vi "Log SPAN autorun Errors.vi"(3 "CompSep":bool, 4 "Sprachliste":string[][](array[string]), 5 "Gasteiler Type":T4 items=["LNI", "Analog-Display", "AVL GDU", "Horiba GDC", "HovaCal", "Horiba SGD 710C"], 6 "Component Infos":T1, 7 "LogFileName_Präfix":string="AutoSpanLin_ErrorLog_", 8 "error in (no error)":errorcluster caption="Fehler (Eingang, kein Fehler)", 9 "LogInfo-Einstellung-Cluster":T5, 10 "LogInfo-Cluster":T6 {"Gasflasche" items=["----"=10000, "IAG NH3 3000"=0, "IAG NH3 200"=1, "IAG NH3 2000"=2, "IAG MG"=3, "IAG O2"=4]}, 11 "Pfad LIN":T8 caption="Pfad") -> (0 "error out":errorcluster caption="Fehler (Ausgang)")   [LabVIEW 2020, in "Linearisierung v2.lvlib" / "SpanEinstellungen.lvlib"]
uses:
  SpanEinstellungen.lvlib
  Visualisierungs Elemente/Pfad-Eingabefeld.ctl
  ErrorLogInfoCluster.ctl
  Visualisierungs Elemente/String - Ausgabefeld.ctl
  Seiten/System Einstellungen V2/Gasflasche Auswahl.ctl
  GasteilerType.ctl
  ComponentInfos.ctl
  Visualisierungs Elemente/String - Eingabefeld.ctl
  Seiten/System Einstellungen V2/Aktion FGV Gasbottledefinition.ctl
  Gasteiler/Aktionen FGV Gasteiler Daten.ctl
  Seiten/System Einstellungen V2/System Einstellungen V2.lvlib
  Gasteiler/Gasteiler.lvlib
  Sprachverwaltung/Sprachverwaltung.lvlib
  Protokoll/Protokoll.lvlib
  Linearisierung v2.lvlib
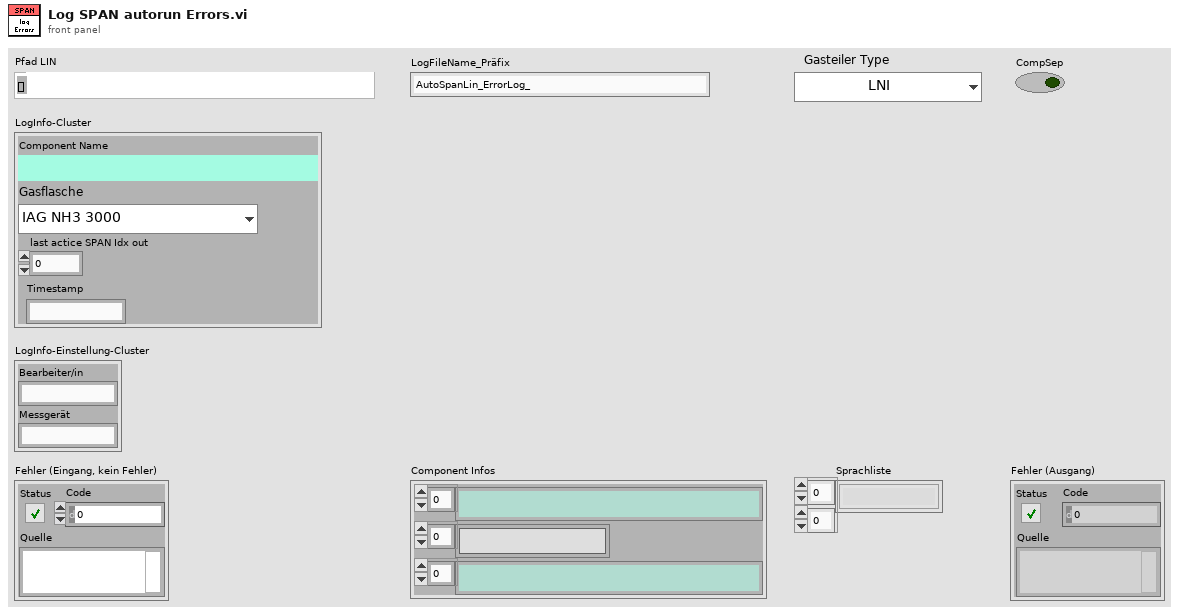
[diagram p1: front panel]
types:
  T1 = typedef "Linearisierung v2.lvlib/SpanEinstellungen.lvlib/ComponentInfos.ctl" = cluster{T2[], T3[], T2[]}
  T2 = typedef "String - Ausgabefeld.ctl" = string
  T3 = typedef "String - Eingabefeld.ctl" = string
  T4 = typedef "Linearisierung v2.lvlib/GasteilerType.ctl" = u16
  T5 = cluster{"Bearbeiter/in":string, "Messgerät":string}
  T6 = typedef "Linearisierung v2.lvlib/SpanEinstellungen.lvlib/ErrorLogInfoCluster.ctl" = cluster{"Component Name":T2, "Gasflasche":T7, "last actice SPAN Idx out":i32, "Timestamp":string}
  T7 = typedef "System Einstellungen V2.lvlib/Gasflasche Auswahl.ctl" = u16
  T8 = typedef "Pfad-Eingabefeld.ctl" = path
  T9 = typedef "Linearisierung v2.lvlib/Gasteiler.lvlib/Aktionen FGV Gasteiler Daten.ctl" = enum16{"lesen", "Gasteiler Daten", "Seriellen Param.", "MB-Endwert", "laden", "speichern", "Anforderung", "TCP", "Aufzeichnung Start"}
  T10 = enum16{"open", "replace", "create", "open or create", "replace or create", "replace or create with confirmation"}
  T11 = typedef "System Einstellungen V2.lvlib/Aktion FGV Gasbottledefinition.ctl" = enum16{"lesen", "schreiben", "löschen", "laden", "speichern", "exportieren", "importieren"}
  T12 = typedef "Linearisierung v2.lvlib/Gasteiler.lvlib/Gasteiler Daten.ctl" = cluster{"Gasteiler":T3, "Gasteiler Stufen":T13, "Gasteiler Type":T4, "Konfig Gasteiler":T14, "Gasteiler Span Eingänge":u16}
  T13 = typedef "Linearisierung v2.lvlib/Gasteiler.lvlib/Gasteiler Stufen.ctl" = u16
  T14 = typedef "System Einstellungen V2.lvlib/Gasteiler Auswahl.ctl" = u16
  T15 = typedef "System Einstellungen V2.lvlib/Gasflasche gesamt.ctl" = cluster{"Gasflasche":T16, "Trägergas":T17, "Komponenten":T18[]}
  T16 = typedef "System Einstellungen V2.lvlib/Gasflasche.ctl" = cluster{"Gasname für die Auswahl":string, "Chargennummer":string, "Ablaufdatum":timestamp}
  T17 = typedef "System Einstellungen V2.lvlib/Traegergas.ctl" = string
  T18 = typedef "System Einstellungen V2.lvlib/Gasflaschenkomponente.ctl" = cluster{"Gasauswahl":string, "Konzentration IST":dbl, "Einheit":string, "Genauigkeit":dbl}
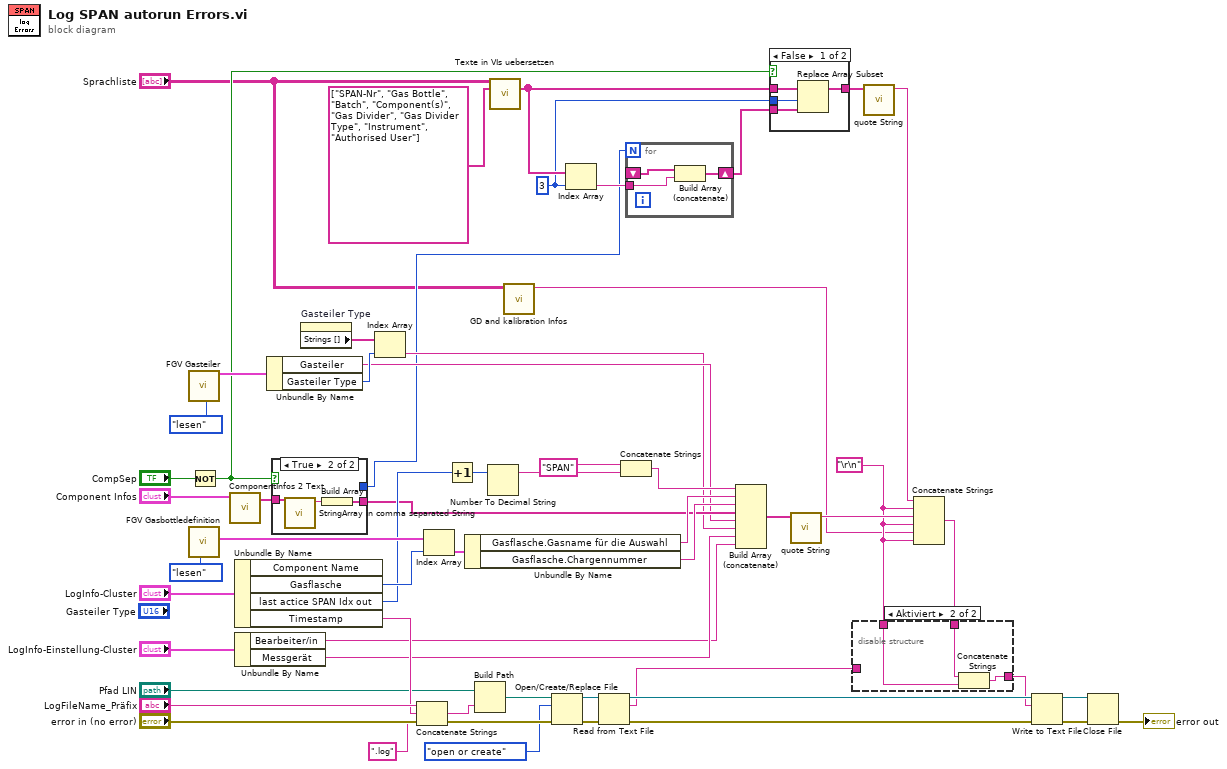
[diagram p0: block diagram]
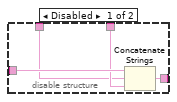
[diagram p2: hidden frame]
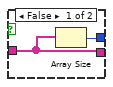
[diagram p3: hidden frame]
diagram:
  w14 = 3 ("Index")
  w7 = "\r\n"
  n1 = call "FGV Gasteiler.vi"("Aktionen"=Aktionen_FGV_Gasteiler_Daten."lesen") -> ("Gasteiler Daten"=w34:T12)  [unwired: 11 in, 7 out]
  n2 = call "FGV Gasbottledefinition.vi"("Aktion"=Aktion_FGV_Gasbottledefinition."lesen") -> ("Gasflaschen Liste gesamt"=w55:T15[])  [unwired: 8 in, 2 out]
  n3 = Not(x="CompSep") -> (.not. x?=w11:bool)
  n4 = call "ComponentInfos 2 Text.vi"("Component Infos"="Component Infos") -> ("Component Text Array"=w3:T2[])  [unwired: 10 in]
  n5 = Unbundle By Name("LogInfo-Cluster") -> ("Gasflasche"=w54:T7, "last actice SPAN Idx out"=w36:i32, "Timestamp"=w51:string)  [unwired: 1 out]
  n6 = Unbundle By Name("LogInfo-Einstellung-Cluster") -> ("Bearbeiter/in"=w20:string, "Messgerät"=w21:string)
  n7 = Unbundle By Name(w34) -> ("Gasteiler"=w23:T3, "Gasteiler Type"=w32:T4)
  n8 = case shown="True" w11 {
    tunnel: w3 -> [w59 w62]
    tunnel: [w59 w60] -> w24
    tunnel: [w58 _] -> w5
    frame False {
      n9 = Array Size(array=w59) -> (size(s)=w58:i32)
    }
    frame True {
      n10 = call "StringArray in comma separated String.vi"("Component Names"=w62) -> ("String"=w61:string)  [unwired: 10 in]
      n11 = Build Array(w61) -> (w60:string[])
    }
  }
  n12 = property on="Gasteiler Type" class="Ring (strikt)"() -> ("Strings []"=w33:string[])  [unwired: 2 in, 2 out]
  n13 = Index Array(array=w33, index=w32) -> (element=w22:string)
  n14 = Concatenate Strings("LogFileName_Präfix", w51, ".log" ("String")) -> (w49:string)
  n15 = Index Array(array=w55, index=w54) -> (element=w53:T15)
  n16 = Increment(x=w36) -> (x+1=w6:i32)
  n17 = Unbundle By Name(w53) -> ("Gasflasche.Gasname für die Auswahl"=w26:string, "Gasflasche.Chargennummer"=w25:string)
  n18 = Build Path(base path="Pfad LIN", name or relative path=w49) -> (appended path=w48:path)
  n19 = Number To Decimal String(number=w6) -> (decimal integer string=w35:string)  [unwired: 1 in]
  n20 = call "Texte in VIs uebersetzen.vi"("Sprachliste"="Sprachliste", "String-Array zum Übersetzen"=string[] ["SPAN-Nr", "Gas Bottle", "Batch", "Component(s)", "Gas Divider", "Gas Divider Type", "Instrument", "Authorised User"]) -> ("String-Array zum Übersetzen"=w17:string[])  [unwired: 9 in, 4 out]
  n21 = call "GD and kalibration Infos.vi"("Sprachliste"="Sprachliste") -> ("ErrorMessages LogFile"=w1:string)  [unwired: 6 in, 4 out]
  n22 = Open/Create/Replace File(file path (use dialog)=w48, error in="error in (no error)", operation (0:open)=T10."open or create" ("Operation (0:open)")) -> (refnum out=w45:refnum<file>, error out=w44:errorcluster)  [unwired: 3 in, 1 out]
  n23 = Index Array(array=w17, index=w14) -> (element=w18:string)
  n24 = Read from Text File(file (use dialog)=w45, error in=w44) -> (refnum out=w43:refnum<file>, text=w10:string, error out=w42:errorcluster)  [unwired: 2 in, 1 out]
  n25 = Concatenate Strings("SPAN", w35) -> (w27:string)
  n26 = for {
    N: w5 -> [_]
    tunnel: w18 -> [w65]
    shift-right: [w64] -> w13
    shift-left: _ -> [w63]
    n27 = Build Array (concatenate)(w63, w65) -> (w64:string[])
  }
  n28 = Build Array (concatenate)(w27, w26, w25, w24, w23, w22, w21, w20) -> (w19:T3[])
  n29 = case shown="False" w11 {
    tunnel: w17 -> [w69 w70]
    tunnel: [w68 w70] -> w15
    tunnel: w14 -> [w67 _]
    tunnel: w13 -> [w66 _]
    frame False {
      n30 = Replace Array Subset(array=w69, new element=w66, index=w67) -> (w68:string[])
    }
    frame True {
    }
  }
  n31 = call "quote String.vi"("String (Eingang)"=w19) -> ("String (Ausgang)"=w29:string)  [unwired: 10 in]
  n32 = call "quote String.vi"("String (Eingang)"=w15) -> ("String (Ausgang)"=w16:string)  [unwired: 10 in]
  n33 = Concatenate Strings(w16, w7, w29, w7, w1, w7) -> (w8:string)
  n34 = disable-structure shown="Aktiviert" {
    disable-tunnel: w10 -> [w74 _]
    disable-tunnel: [w73 w76] -> w9
    disable-tunnel: w8 -> [w72 w77]
    disable-tunnel: w7 -> [w71 w75]
    frame Disabled {
      n35 = Concatenate Strings(w74, w71, w72) -> (w73:string)
    }
    frame Enabled {
      n36 = Concatenate Strings(w77, w75) -> (w76:string)
    }
  }
  n37 = Write to Text File(file (use dialog)=w43, text=w9, error in=w42) -> (refnum out=w40:refnum<file>, error out=w41:errorcluster)  [unwired: 1 in, 1 out]
  n38 = Close File(refnum=w40, error in=w41) -> (error out=→"error out":errorcluster)  [unwired: 1 out]
